vi "Compass Constructor.vi"(8 "error in (no error)":errorcluster, 9 "radius vector":dbl[](array[numeric]), 10 "theta vector":dbl[](array[numeric]), 11 "2D Compass Datatype.lvclass in":refnum<class "2D Compass Datatype.lvclass">) -> (0 "error out":errorcluster, 3 "2D Compass Datatype.lvclass out":refnum<class "2D Compass Datatype.lvclass">)   [LabVIEW 2017, in "2D Compass Datatype.lvclass"]
uses:
  <vilib>/Math Plots/2D Math Plots/2D Compass/2D Compass Datatype/2D Compass Datatype.lvclass
  <vilib>/Math Plots/2D Math Plots/2D Compass/2D Compass Datatype/2D Compass Datatype.lvclass/2D Compass Datatype.ctl
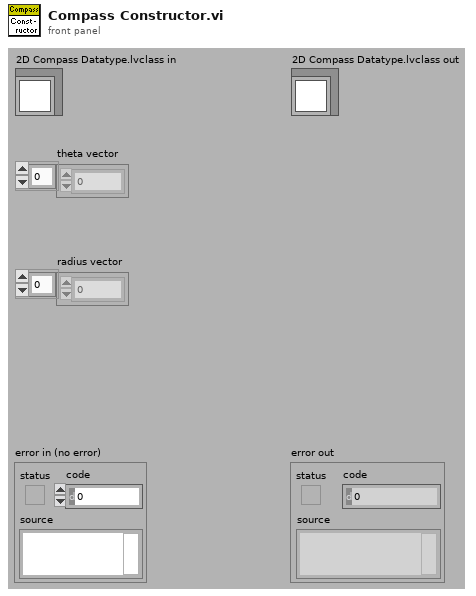
[diagram p1: front panel]
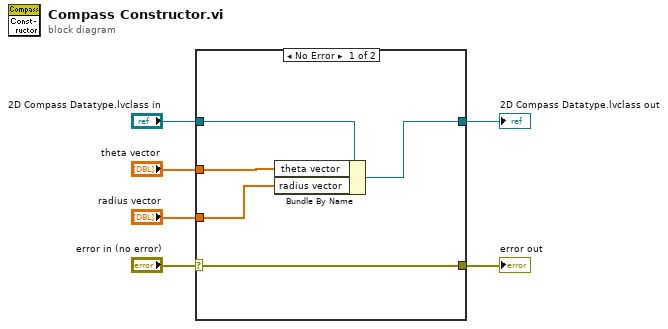
[diagram p0: block diagram]
diagram:
  n1 = case shown="No Error" "error in (no error)" {
    selector: "error in (no error)" -> [w11 w13]
    tunnel: [w11 w13] -> w2
    tunnel: "theta vector" -> [w9 _]
    tunnel: "radius vector" -> [w8 _]
    tunnel: "2D Compass Datatype.lvclass in" -> [w10 w12]
    tunnel: [w7 w12] -> w6
    frame No Error {
      n2 = Bundle By Name(cluster=w10, "theta vector"=w9, "radius vector"=w8) -> (w7:refnum<class "2D Compass Datatype.lvclass">)
    }
    frame Error {
    }
  }
  "error out" <- w2
  "2D Compass Datatype.lvclass out" <- w6
